vi "hysteresis.vi"(1 "Size":dbl, 2 "In":dbl) -> (0 "Out":dbl)   [LabVIEW 2023]
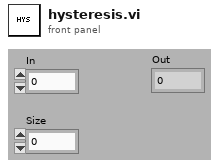
[diagram p1: front panel]
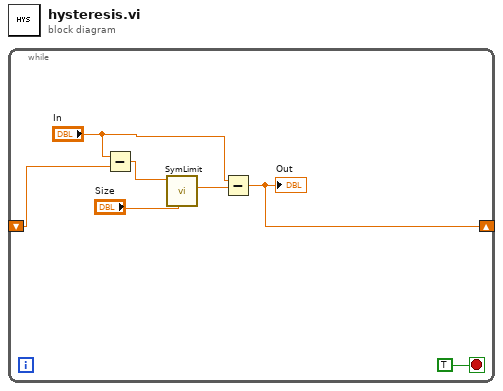
[diagram p0: block diagram]
diagram:
  n1 = while {
    shift-right: [w6] -> _
    shift-left: _ -> [w4]
    stop <- TRUE stop-if-true
    n2 = Subtract(x="In", y=w4) -> (x-y=w3:dbl)
    n3 = call "SymLimit.vi"("Limit"="Size", "Input"=w3) -> ("Output"=w1:dbl)  [unwired: 9 in]
    n4 = Subtract(x="In", y=w1) -> (x-y=w6:dbl)
    "Out" <- w6
  }
